vi "Create_setup_string.vi"() -> (0 "Setup String":string)   [LabVIEW 2021]
uses:
  Globals/Meas_global.vi
  Globals/Trav_pos_global.vi
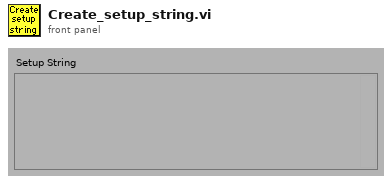
[diagram p1: front panel]
types:
  T1 = typedef "Analysis_info_cluster.ctl" = cluster{"Colour":u32, "Inst type":T2, "Inst name":string, "Symbol":string, "Code name":string, "Extra Info":string, "Inst Array":T3, "Extra Titles":string[], "Extra Values":string[], "U":dbl, "u^2":dbl, "u^3":dbl, "u^4":dbl, "Skew_u":dbl, "Kurt_u":dbl, "Sd Error in Mean":dbl, "% u'/U":dbl, "X":dbl, "Y":dbl, "Z":dbl, "Timescale integral Estimate":dbl, "Sd Error in Variance":dbl, "Calib File":path, "Calib Constants":dbl[], "Output Position":bool, "Stats":enum16{"None", "Basic", "Full"}, "Av Sampling Rate":dbl, "Av No of Samples":dbl, "Total Meas Time (s)":dbl, "ADAM Ch Name":string, "Max value":dbl, "Min value":dbl, "Req Sample Rate Hz":dbl, "Sync Delay Time (s)":dbl, "Ch No":i16, "Device":string, "Use Latest Calib":bool, "Port":string, "Metadata Ch Names":string[], "Metadata Ch Values":string[], "Label":string}
  T2 = typedef "Inst_type.ctl" = enum16{"Raw voltage", "Raw with zero offsetting", "Propeller anemometer", "Pressure Transducer", "Pitot-static tube", "Hot wire", "Cross wire 1", "Cross wire 2", "Generic Linear", "Generic Polynomial", "Generic BackPoly", "Fast FID", "Thermocouple", "Cold wire", "Pulsed Wire", "LDA Vel", "LDA Tran time", "LDA Arr time", "Microphone"}
  T3 = typedef "Instrument_Array.ctl" = enum16{"PWA", "LDA", "Analogue"}
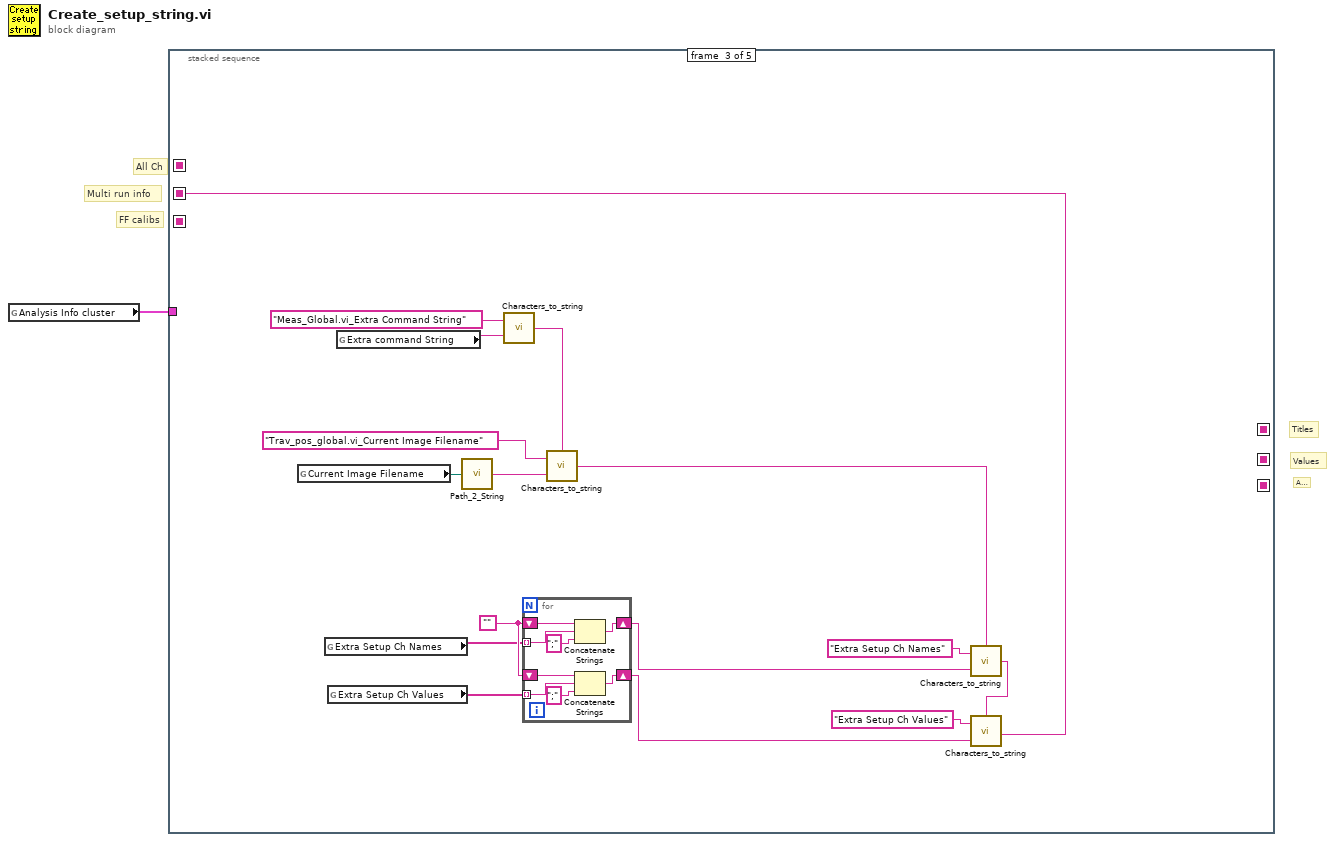
[diagram p0: block diagram]
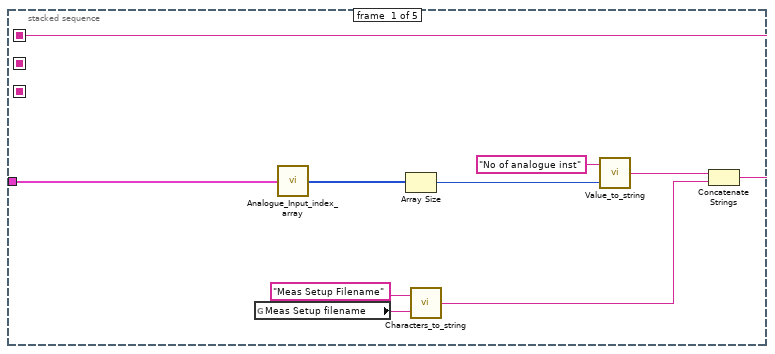
[diagram p2: hidden frame]
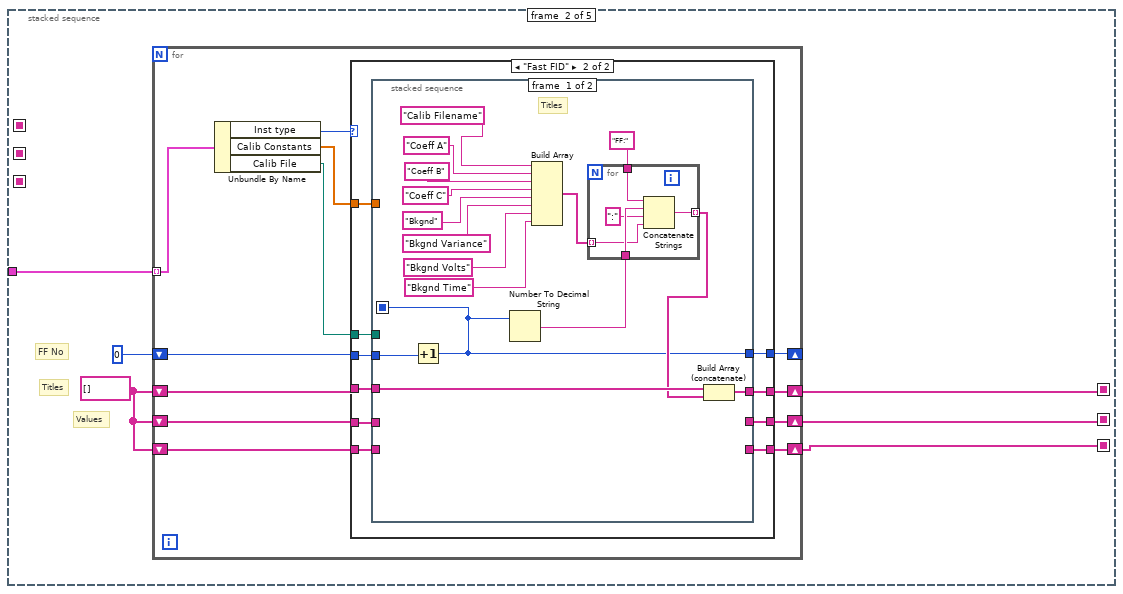
[diagram p3: hidden frame]
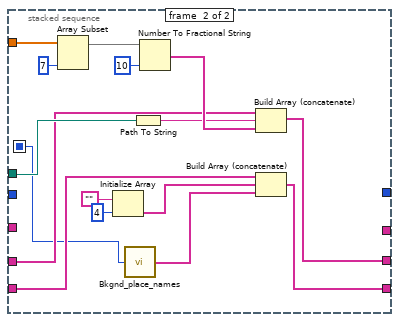
[diagram p5: hidden frame]
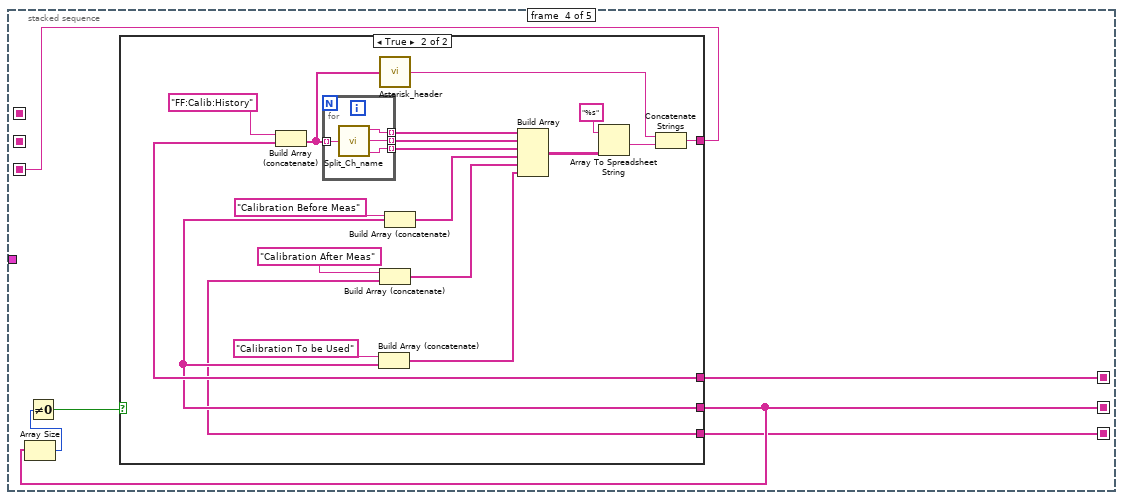
[diagram p6: hidden frame]
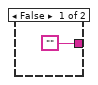
[diagram p7: hidden frame]
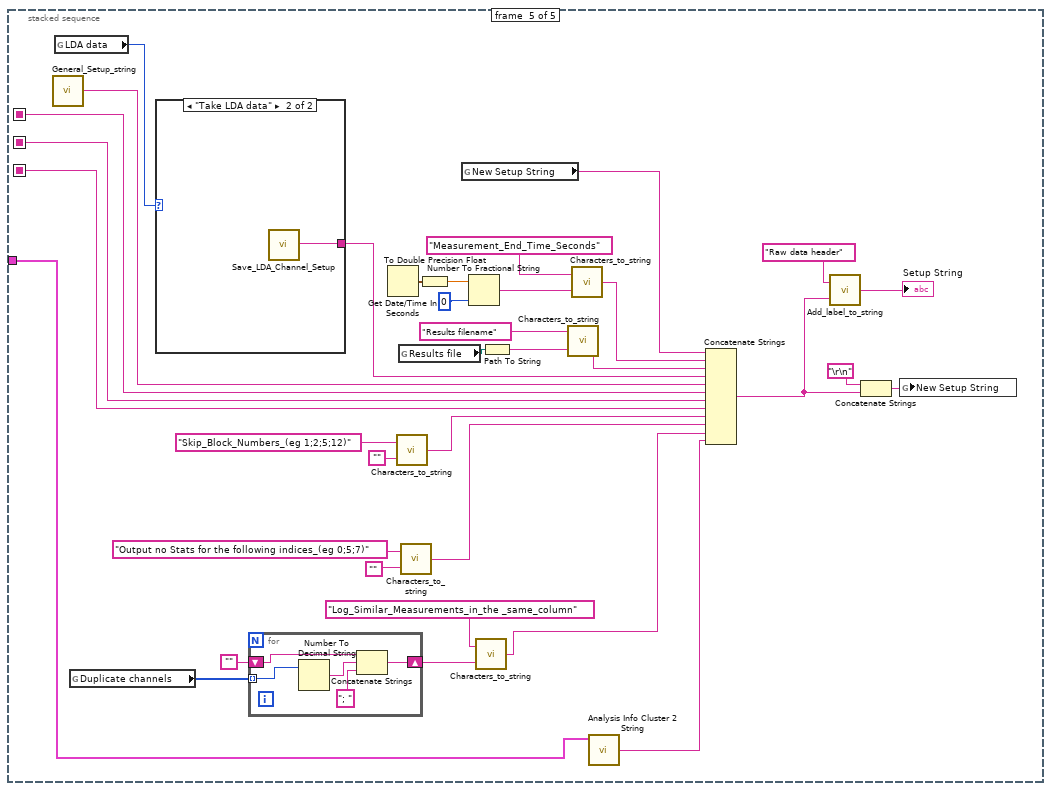
[diagram p8: hidden frame]
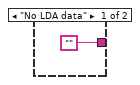
[diagram p9: hidden frame]
diagram:
  # "Multi run info"
  # "After"
  # "Values"
  # "Titles"
  # "FF calibs"
  # "All Ch"
  n1 = global read "Meas_global.vi" "Analysis Info cluster"() -> (w1:T1[])
  n2 = stacked-sequence {
    seq-local: [w8 _ _ _ _] -> [_ _ _ _ w168]
    seq-local: [_ _ _ w108 _] -> [_ _ _ _ w148]
    seq-local: [_ w14 _ _ _] -> [_ _ _ w109 _]
    seq-local: [_ w15 _ _ _] -> [_ _ _ w106 _]
    seq-local: [_ w12 _ _ _] -> [_ _ _ w104 _]
    seq-local: [_ _ w80 _ _] -> [_ _ _ _ w147]
    tunnel: w1 -> [w5 w11 _ _ w140]
    frame #0 {
      n3 = global read "Meas_global.vi" "Meas Setup filename"() -> (w4:string)
      n4 = call "Analogue_Input_index_array.vi"("Analysis Info cluster"=w5) -> ("Array"=w6:i32[])
      n5 = Array Size(array=w6) -> (size(s)=w7:i32)
      n6 = call "Characters_to_string.vi"("Characters to write"=w4, "Label for characters"="Meas Setup Filename") -> ("Output string"=w2:string)  [unwired: 1 in]
      n7 = call "Value_to_string.vi"("Value"=w7, "Label for value"="No of analogue inst") -> ("Output string"=w9:string)  [unwired: 1 in]
      n8 = Concatenate Strings(w9, w2) -> (w8:string)
    }
    frame #1 {
      w13 = string[] []
      # "Values"
      # "Titles"
      # "FF No"
      n9 = for {
        shift-right: [w24] -> w14
        shift-left: w13 -> [w25]
        shift-right: [w26] -> _
        shift-left: 0 -> [w27]
        shift-right: [w22] -> w15
        shift-left: w13 -> [w23]
        shift-right: [w20] -> w12
        shift-left: w13 -> [w21]
        tunnel: w11 -> [w17] mode=indexing
        n10 = Unbundle By Name(w17) -> ("Inst type"=w28:T2, "Calib Constants"=w19:dbl[], "Calib File"=w18:path)
        n11 = case shown="\"Fast FID\"" w28 {
          tunnel: w19 -> [_ w42]
          tunnel: w18 -> [_ w41]
          tunnel: w27 -> [w32 w40]
          tunnel: [w32 w39] -> w26
          tunnel: w25 -> [w31 w38]
          tunnel: [w31 w37] -> w24
          tunnel: w23 -> [w30 w36]
          tunnel: [w30 w35] -> w22
          tunnel: w21 -> [w29 w34]
          tunnel: [w29 w33] -> w20
          frame "Propeller anemometer", Default {
          }
          frame "Fast FID" {
            n12 = stacked-sequence {
              seq-local: [w43 _] -> [_ w65]
              tunnel: w42 -> [_ w78]
              tunnel: w41 -> [_ w79]
              tunnel: w40 -> [w58 _]
              tunnel: [w43 _] -> w39
              tunnel: w38 -> [w54 _]
              tunnel: [w53 _] -> w37
              tunnel: w36 -> [_ w73]
              tunnel: [_ w72] -> w35
              tunnel: w34 -> [_ w70]
              tunnel: [_ w69] -> w33
              frame #0 {
                # "Titles"
                n13 = Increment(x=w58) -> (x+1=w43:i32)
                n14 = Number To Decimal String(number=w43) -> (decimal integer string=w44:string)  [unwired: 1 out]
                n15 = Build Array("Calib Filename", "Coeff A", "Coeff B", "Coeff C", "Bkgnd", "Bkgnd Variance", "Bkgnd Volts", "Bkgnd Time") -> (w55:string[])
                n16 = for {
                  tunnel: "FF:" -> [w63]
                  tunnel: w44 -> [w62]
                  tunnel: w55 -> [w60] mode=indexing
                  tunnel: [w59] -> w47 mode=indexing
                  n17 = Concatenate Strings(w63, w62, ":" ("Substring"), w60) -> (w59:string)
                }
                n18 = Build Array (concatenate)(w54, w47) -> (w53:string[])
              }
              frame #1 {
                n19 = Array Subset(array=w78, length=7 ("Array Length")) -> (w76:dbl[])  [unwired: 1 in]
                n20 = Initialize Array("", 4 ("dimension size")) -> (w66:string[])
                n21 = call "Bkgnd_place_names.vi"("Numeric"=w65) -> ("Array"=w64:string[])
                n22 = Path To String(path=w79) -> (string=w71:string)
                n23 = Number To Fractional String(number=w76, precision (6)=i16 10) -> (F-format string=w74:string[])  [unwired: 2 out]
                n24 = Build Array (concatenate)(w73, w71, w74) -> (w72:string[])
                n25 = Build Array (concatenate)(w70, w66, w64) -> (w69:string[])
              }
            }
          }
        }
      }
    }
    frame #2 {
      w87 = ""
      n26 = global read "Trav_pos_global.vi" "Current Image Filename"() -> (w93:path)
      n27 = global read "Meas_global.vi" "Extra Setup Ch Names"() -> (w86:string[])
      n28 = global read "Meas_global.vi" "Extra Setup Ch Values"() -> (w85:string[])
      n29 = global read "Meas_global.vi" "Extra command String"() -> (w95:string)
      n30 = call "Path_2_String.vi"("Real Path"=w93) -> ("Path String"=w92:string)
      n31 = call "Characters_to_string.vi"("Characters to write"=w95, "Label for characters"="Meas_Global.vi_Extra Command String") -> ("Output string"=w90:string)  [unwired: 1 in]
      n32 = for {
        shift-right: [w102] -> w84
        shift-left: w87 -> [w103]
        tunnel: w86 -> [w98] mode=indexing
        shift-right: [w101] -> w83
        shift-left: w87 -> [w99]
        tunnel: w85 -> [w100] mode=indexing
        n33 = Concatenate Strings(w103, w98, ";" ("string")) -> (w102:string)
        n34 = Concatenate Strings(w99, w100, ";" ("string")) -> (w101:string)
      }
      n35 = call "Characters_to_string.vi"("stringIn"=w90, "Characters to write"=w92, "Label for characters"="Trav_pos_global.vi_Current Image Filename") -> ("Output string"=w82:string)
      n36 = call "Characters_to_string.vi"("stringIn"=w82, "Characters to write"=w84, "Label for characters"="Extra Setup Ch Names" ("Variable name")) -> ("Output string"=w81:string)
      n37 = call "Characters_to_string.vi"("stringIn"=w81, "Characters to write"=w83, "Label for characters"="Extra Setup Ch Values" ("Variable name")) -> ("Output string"=w80:string)
    }
    frame #3 {
      n38 = Array Size(array=w106) -> (size(s)=w107:i32)
      n39 = Not Equal To 0?(x=w107) -> (x != 0?=w105:bool)
      n40 = case shown="True" w105 {
        tunnel: w109 -> [_ w126]
        tunnel: w106 -> [_ w120]
        tunnel: ["" w114] -> w108
        tunnel: w104 -> [_ w112]
        frame False {
        }
        frame True {
          n41 = Build Array (concatenate)("FF:Calib:History" ("Input Element"), w126) -> (w117:string[])
          n42 = for {
            tunnel: w117 -> [w133] mode=indexing
            tunnel: [w132] -> w129 mode=indexing
            tunnel: [w131] -> w128 mode=indexing
            tunnel: [w130] -> w127 mode=indexing
            n43 = call "Split_Ch_name.vi"("Ch name"=w133) -> ("Top level"=w132:string, "Middle"=w131:string, "Low level"=w130:string)
          }
          n44 = Build Array (concatenate)("Calibration To be Used" ("Input Element"), w120) -> (w122:string[])
          n45 = call "Asterisk_header.vi"("Channel names"=w117) -> ("Header string"=w115:string)
          n46 = Build Array (concatenate)("Calibration After Meas" ("Input Element"), w112) -> (w111:string[])
          n47 = Build Array (concatenate)("Calibration Before Meas" ("Input Element"), w120) -> (w123:string[])
          n48 = Build Array(w129, w128, w127, w123, w111, w122) -> (w118:string[][])
          n49 = Array To Spreadsheet String(array=w118, 3:"%s" ("format string")) -> (spreadsheet string=w116:string)  [unwired: 1 out]
          n50 = Concatenate Strings(w115, w116) -> (w114:string)
        }
      }
    }
    frame #4 {
      n51 = call "General_Setup_string.vi"() -> ("Output string"=w141:string)  [unwired: 1 out]
      n52 = global read "Meas_global.vi" "LDA data"() -> (w143:enum16{"No LDA data", "Take LDA data"})
      n53 = global read "Meas_global.vi" "Duplicate channels"() -> (w136:i32[])
      n54 = case shown="\"Take LDA data\"" w143 {
        tunnel: ["" w175] -> w142
        frame "No LDA data" {
        }
        frame "Take LDA data" {
          n55 = call "Save_LDA_Channel_Setup.vi"() -> ("Setup file string"=w175:string)  [unwired: 1 in]
        }
      }
      n56 = for {
        shift-right: [w169] -> w138
        shift-left: "" -> [w172]
        tunnel: w136 -> [w173] mode=indexing
        n57 = Number To Decimal String(number=w173) -> (decimal integer string=w171:string)  [unwired: 1 out]
        n58 = Concatenate Strings(w172, w171, "; ") -> (w169:string)
      }
      n59 = Get Date/Time In Seconds() -> (seconds since 1Jan1904=w156:timestamp)
      n60 = call "Characters_to_string.vi"("Characters to write"="", "Label for characters"="Skip_Block_Numbers_(eg 1;2;5;12)" ("Variable name")) -> ("Output string"=w150:string)  [unwired: 1 in]
      n61 = global read "Meas_global.vi" "Results file"() -> (w165:path)
      n62 = call "Characters_to_string.vi"("Characters to write"="", "Label for characters"="Output no Stats for the following indices_(eg 0;5;7)" ("Variable name")) -> ("Output string"=w144:string)  [unwired: 1 in]
      n63 = To Double Precision Float(number=w156) -> (double precision float=w158:dbl)
      n64 = global read "Meas_global.vi" "New Setup String"() -> (w149:string)
      n65 = Number To Fractional String(number=w158, precision (6)=i16 0) -> (F-format string=w155:string)  [unwired: 2 out]
      n66 = call "Characters_to_string.vi"("Characters to write"=w138, "Label for characters"="Log_Similar_Measurements_in_the _same_column") -> ("Output string"=w135:string)  [unwired: 1 in]
      n67 = Path To String(path=w165) -> (string=w162:string)
      n68 = call "Characters_to_string.vi"("Characters to write"=w162, "Label for characters"="Results filename") -> ("Output string"=w166:string)  [unwired: 1 in]
      n69 = call "Characters_to_string.vi"("Characters to write"=w155, "Label for characters"="Measurement_End_Time_Seconds") -> ("Output string"=w153:string)  [unwired: 1 in]
      n70 = call "Analysis Info Cluster 2 String.vi"("Analysis Info cluster"=w140) -> ("Output string"=w134:string)  [unwired: 5 in]
      n71 = Concatenate Strings(w149, w153, w166, w142, w141, w168, w147, w148, w150, w144, w135, w134) -> (w160:string)
      n72 = call "Add_label_to_string.vi"("String to write"=w160, "File Label"="Raw data header") -> ("Output string"=→"Setup String":string)
      n73 = Concatenate Strings("\r\n", w160) -> (w161:string)
      n74 = global write "Meas_global.vi" "New Setup String"(w161) -> ()
    }
  }
